vi "MorseCodeParser.vi"() -> ()   [LabVIEW 2018]
panel:
  out "String Output":string
  in  "Within a letter":string="/"
  out "Array 2":string[](array[string])
  in  "Within word":string="///"
  in  "Spaces":string="///////"
  out "Array":string[][][](array[string])
  in  "String":string
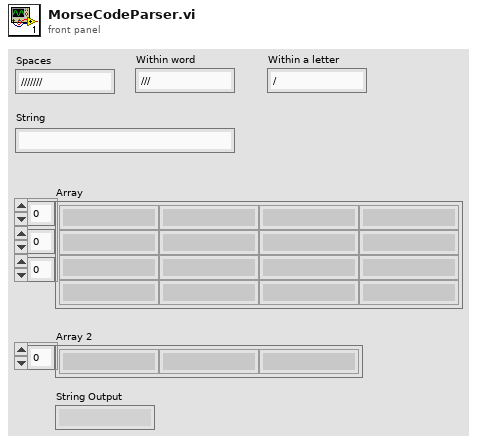
[diagram p1: front panel]
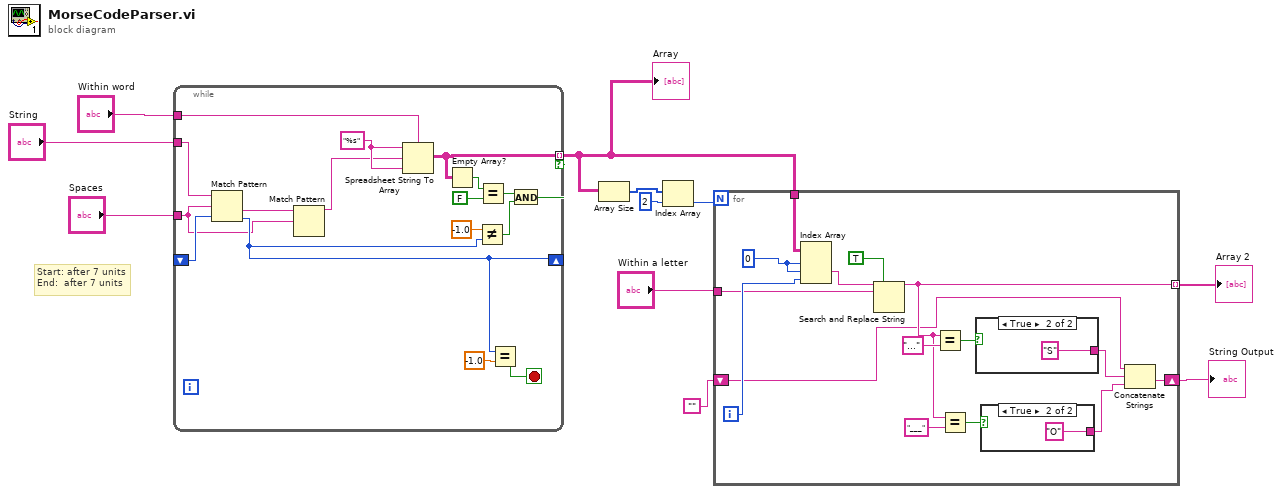
[diagram p0: block diagram]
diagram:
  # "Start: after 7 units\nEnd:  after 7 units"
  n1 = while {
    tunnel: "String" -> [w28]
    shift-right: [w22] -> _
    shift-left: _ -> [w27]
    tunnel: [w12] -> w5 mode=indexing if=w19
    tunnel: "Spaces" -> [w14]
    tunnel: "Within word" -> [w13]
    stop <- w26 stop-if-true
    w18 = "%s" ("format string")
    n2 = Match Pattern(string=w28, regular expression=w14, offset (0)=w27) -> (after substring=w17:string, offset past match=w22:i32)  [unwired: 2 out]
    n3 = Match Pattern(string=w17, regular expression=w14) -> (before substring=w16:string)  [unwired: 1 in, 3 out]
    n4 = Spreadsheet String To Array(delimiter (Tab)=w13, format string=w18, spreadsheet string=w16, array type (2D Dbl)=w18) -> (array=w12:string[][])
    n5 = Empty Array?(array=w12) -> (empty?=w15:bool)
    n6 = Not Equal?(x=-1.0, y=w22) -> (x != y?=w20:bool)
    n7 = Equal?(x=w15, y=FALSE) -> (x = y?=w21:bool)
    n8 = Equal?(x=w22, y=-1.0) -> (x = y?=w26:bool)
    n9 = And(x=w21, y=w20) -> (x .and. y?=w19:bool)
  }
  "Array" <- w5
  n10 = Array Size(array=w5) -> (size(s)=w8:i32[])
  n11 = Index Array(array=w8, index=2) -> (element=w6:i32)
  n12 = for {
    N: w6 -> [_]
    tunnel: w5 -> [w43]
    tunnel: [w34] -> w4 mode=indexing
    tunnel: "Within a letter" -> [w38]
    shift-right: [w32] -> w1
    shift-left: "" -> [w29]
    i -> [w42]
    w41 = 0 ("disabled index (page)")
    n13 = Index Array(array=w43, index (dim 0)=w41, index (dim 1)=w41, index (dim 2)=w42) -> (element=w40:string)
    n14 = Search and Replace String(replace all?=TRUE ("replace all? (F)"), input string=w40, search string=w38) -> (result string=w34:string)  [unwired: 5 in, 3 out]
    n15 = Equal?(x=w34, y="...") -> (x = y?=w37:bool)
    n16 = Equal?(x=w34, y="___") -> (x = y?=w36:bool)
    n17 = case shown="True" w37 {
      tunnel: [_ "S"] -> w30
      frame False {
      }
      frame True {
      }
    }
    n18 = case shown="True" w36 {
      tunnel: [_ "O"] -> w31
      frame False {
      }
      frame True {
      }
    }
    n19 = Concatenate Strings(w29, w30, w31) -> (w32:string)
  }
  "Array 2" <- w4
  "String Output" <- w1
